vi "RTS Defrost To Defrost kWh.vi"(8 "Error In":errorcluster, 11 "Refrigeration Core Stats":T1 {"Average Compressor Cycle Time (Min)" format="%0.2f"; "Average Compressor Power (W)" format="%0.2f"; "Power Start Time (sec)" format="%<%H:%M:%S>t"; "Power End time (sec)" format="%<%H:%M:%S>t"; "Average Defrost Power (W)" format="%0.2f"}) -> (0 "Error Out":errorcluster, 3 "Refrigeration Core Stats Out":T1 {"Average Compressor Cycle Time (Min)" format="%0.2f"; "Average Compressor Power (W)" format="%0.2f"; "Power Start Time (sec)" format="%<%H:%M:%S>t"; "Power End time (sec)" format="%<%H:%M:%S>t"; "Average Defrost Power (W)" format="%0.2f"})   [LabVIEW 2016]
uses:
  Type Definitions/RTS Macro Refrigeration Core Stats.ctl
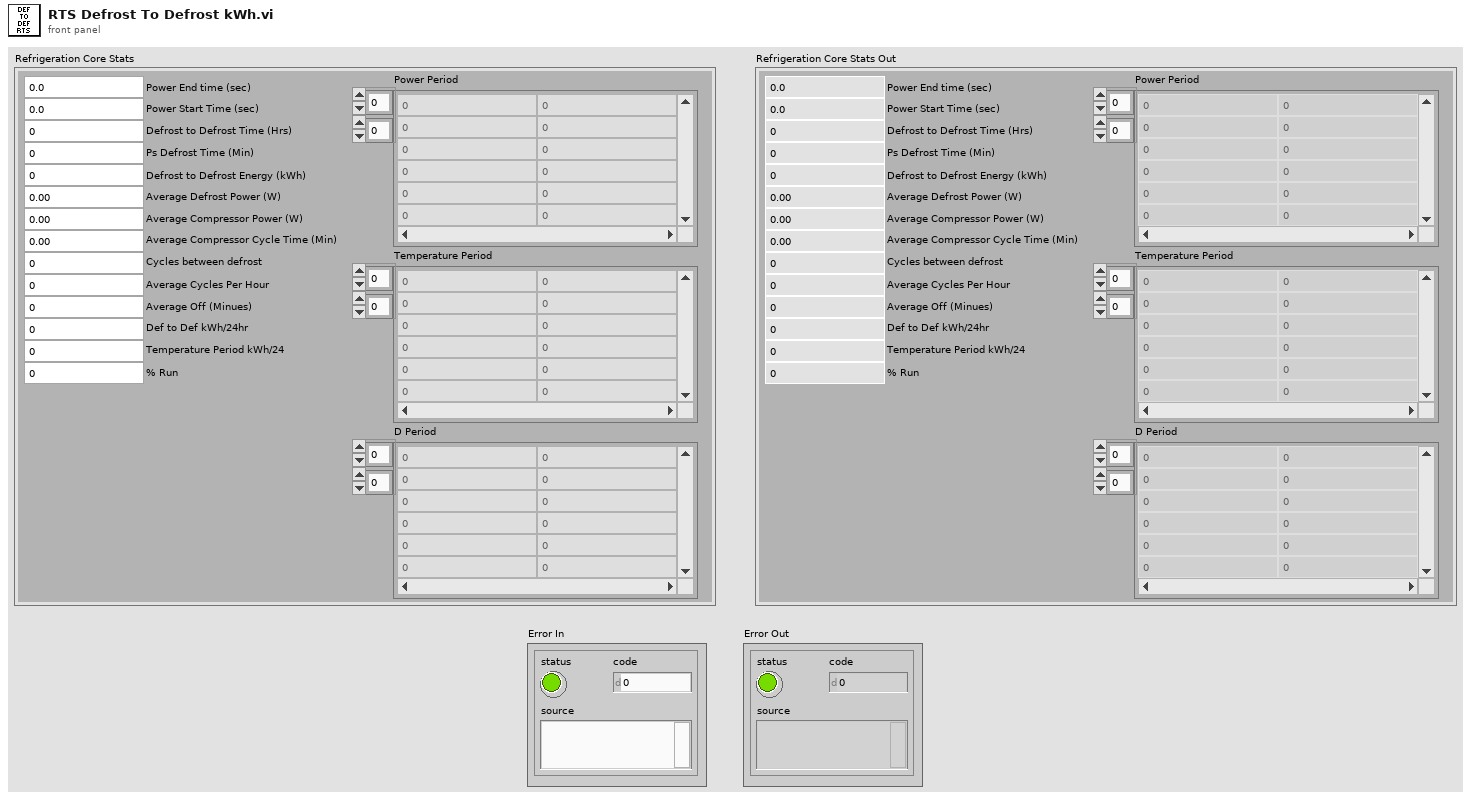
[diagram p1: front panel]
types:
  T1 = typedef "RTS Macro Refrigeration Core Stats.ctl" = cluster{"Average Defrost Power (W)":dbl, "Power End time (sec)":dbl, "Power Start Time (sec)":dbl, "Defrost to Defrost Time (Hrs)":dbl, "Ps Defrost Time (Min)":dbl, "Defrost to Defrost Energy (kWh)":dbl, "Average Compressor Power (W)":dbl, "Average Compressor Cycle Time (Min)":dbl, "Power Period":dbl[][], "Cycles between defrost":i32, "Average Cycles Per Hour":dbl, "Average Off (Minues)":dbl, "Def to Def kWh/24hr":dbl, "Temperature Period kWh/24":dbl, "% Run":dbl, "Temperature Period":dbl[][], "D Period":dbl[][]}
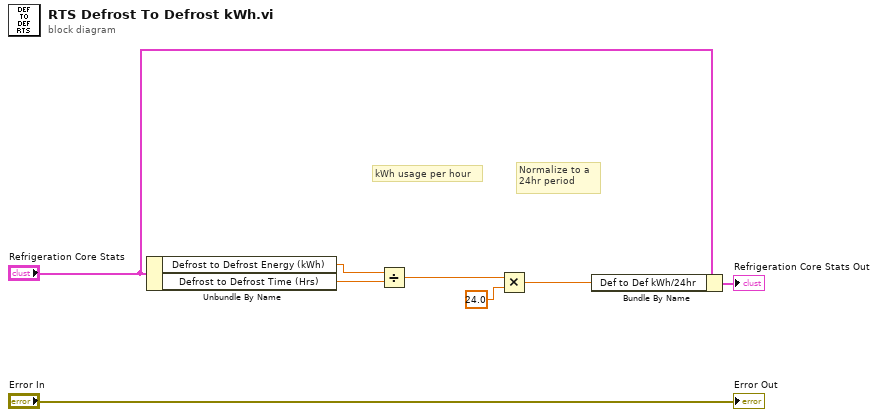
[diagram p0: block diagram]
diagram:
  # "Normalize to a \n24hr period"
  # "kWh usage per hour"
  n1 = Unbundle By Name("Refrigeration Core Stats") -> ("Defrost to Defrost Energy (kWh)"=w5:dbl, "Defrost to Defrost Time (Hrs)"=w4:dbl)
  n2 = Divide(x=w5, y=w4) -> (x/y=w3:dbl)
  n3 = Multiply(x=w3, y=24.0) -> (x*y=w1:dbl)
  n4 = Bundle By Name(cluster="Refrigeration Core Stats", "Def to Def kWh/24hr"=w1) -> (→"Refrigeration Core Stats Out":T1)
  "Error Out" <- "Error In"
